vi "generateName.vi"() -> (2 "buffername":string)   [LabVIEW 2016]
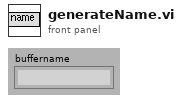
[diagram p1: front panel]
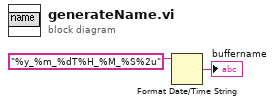
[diagram p0: block diagram]
diagram:
  n1 = Format Date/Time String(time format string (%c)="%y_%m_%dT%H_%M_%S%2u") -> (date/time string=→"buffername":string)  [unwired: 2 out]
